vi "Test Positive Definite (DBL).vi"(10 "relative tolerance":dbl=-1.0, 11 "Input Matrix":T1) -> (0 "error":i32, 3 "positive definite?":bool)   [LabVIEW 2020, in "NI_AALPro.lvlib"]
uses:
  <vilib>/Analysis/NI_AALPro.lvlib
  <vilib>/Analysis/Matrix/Datatypes/RealMatrix.ctl
  <resource>/lvanlys.dll
  <vilib>/Analysis/Matrix/NI_Matrix.lvlib
panel:
  # "Test Positive Definite"
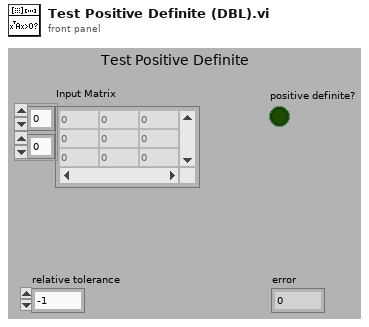
[diagram p1: front panel]
types:
  T1 = typedef "NI_Matrix.lvlib/RealMatrix.ctl" = dbl[][]
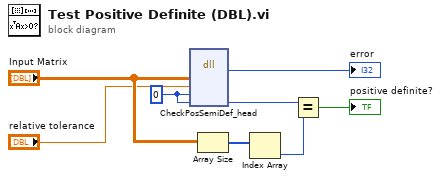
[diagram p0: block diagram]
diagram:
  w4 = 0 ("_possemidef")
  n1 = dll-call lib="e:/builds/penguin/labview/branches/2020/dev/dist/resource/lvanlys.*" fn="CheckPosSemiDef_head"("_aH"="Input Matrix", "_tol"="relative tolerance", "_possemidef"=w4, "_rank"=w4) -> ("return type"=→"error":i32, "_rank"=w3:i32)  [unwired: 6 in, 2 out]
  n2 = Array Size(array="Input Matrix") -> (size(s)=w2:i32[])
  n3 = Index Array(array=w2) -> (element=w1:i32)  [unwired: 1 in]
  n4 = Equal?(x=w3, y=w1) -> (x = y?=→"positive definite?":bool)
